vi "Check If Line Exists.vi"(8 "error in":errorcluster, 10 "name to locate":string, 11 "OPC UA configuration in":refnum<class "OPC UA Client configuration.lvclass">) -> (0 "error out":errorcluster, 1 "index":i32, 2 "Line out":T1 {"OPC UA Data Type" items=["Boolean"=1, "SByte"=2, "Byte"=3, "Int16"=4, "UInt16"=5, "Int32"=6, "UInt32"=7, "Int64"=8, "UInt64"=9, "Float"=10, "Double"=11, "String"=12, "DateTime"=13, "ByteString"=15, "Array of Boolean"=101, "Array of SByte"=102, "Array of Byte"=103, "Array of Int16"=104, "Array of UInt16"=105, "Array of Int32"=106, "Array of UInt32"=107, "Array of Int64"=108, "Array of UInt64"=109, "Array of Float"=110, "Array of Double"=111, "Array of String"=112, "Array of DateTime"=113, "Array of ByteString"=115]}, 3 "OPC UA configuration out":refnum<class "OPC UA Client configuration.lvclass">, 5 "found?":bool)   [LabVIEW 2014, in "OPC UA Client configuration.lvclass"]
uses:
  OPC UA Client configuration.lvclass
  Line.ctl
  <vilib>/NI/Tag Bus Module Framework/channel/TBM channel.lvclass
  OPC UA Data Type.ctl
  OPC UA Client configuration.lvclass/OPC UA Client configuration.ctl
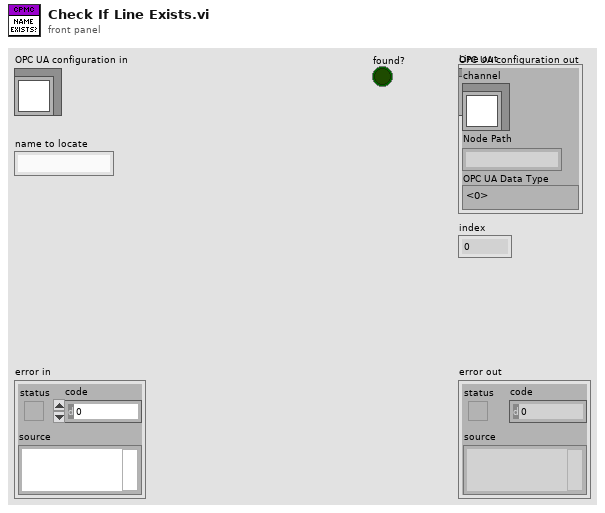
[diagram p1: front panel]
types:
  T1 = typedef "OPC UA Client configuration.lvclass/Line.ctl" = cluster{"channel":refnum<class "TBM channel.lvclass">, "Node Path":string, "OPC UA Data Type":T2}
  T2 = typedef "OPC UA Client configuration.lvclass/OPC UA Data Type.ctl" = u16
  T3 = cluster{"channel":refnum<class "TBM channel.lvclass">, "Node Path":string, "OPC UA Data Type":T2}[]
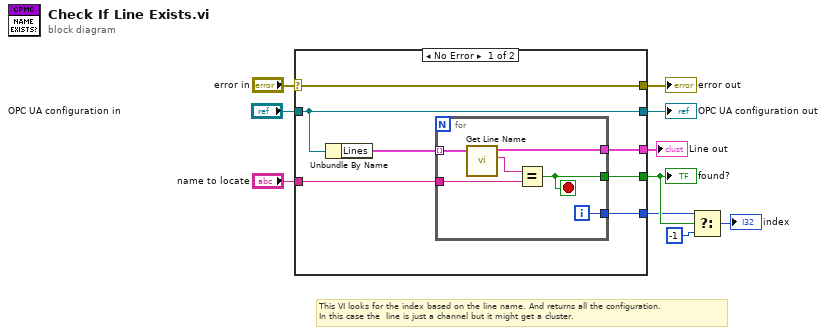
[diagram p0: block diagram]
diagram:
  # "This VI looks for the index based on the line name. And returns all the configuration. \nIn this case the  line is just a channel but it might get a cluster."
  n1 = case shown="No Error" "error in" {
    selector: "error in" -> [w17 w25]
    tunnel: [w17 w25] -> w9
    tunnel: [w16 w24] -> w7
    tunnel: "OPC UA configuration in" -> [w16 w24]
    tunnel: "name to locate" -> [w14 _]
    tunnel: [w13 _] -> w3
    tunnel: [w12 _] -> w2
    tunnel: [w11 _] -> w1
    frame No Error {
      n2 = Unbundle By Name(w16) -> ("Lines"=w15:T3)
      n3 = for {
        tunnel: w15 -> [w20] mode=indexing
        tunnel: w14 -> [w23]
        tunnel: [w22] -> w13
        tunnel: [w21] -> w12
        tunnel: [w18] -> w11
        i -> [w21]
        stop <- w22 stop-if-true
        n4 = call "Get Line Name.vi"("Line in"=w20) -> ("Name"=w19:string, "Line out"=w18:T1)  [unwired: 8 in, 1 out]
        n5 = Equal?(x=w19, y=w23) -> (x = y?=w22:bool)
      }
    }
    frame Error {
    }
  }
  "error out" <- w9
  "OPC UA configuration out" <- w7
  "found?" <- w3
  "Line out" <- w1
  n6 = Select(t=w2, s=w3, f=-1) -> (s? t:f=→"index":i32)
